vi "Koinzidenzschaltung.vi"() -> ()   [LabVIEW 2024]
panel:
  in  "Abbrechen":bool
  in  "Measunring Time (ms)":dbl max=0.0 step=10.0
  in  "StepSize (mV)":dbl max=0.0 step=10.0
  in  "Stop Value (mV)":dbl max=0.0 step=10.0
  out "Current Value":dbl
  in  "Start Value (mV)":dbl max=0.0 step=10.0
  out "Versoion":string
  out "NemBox ID":string
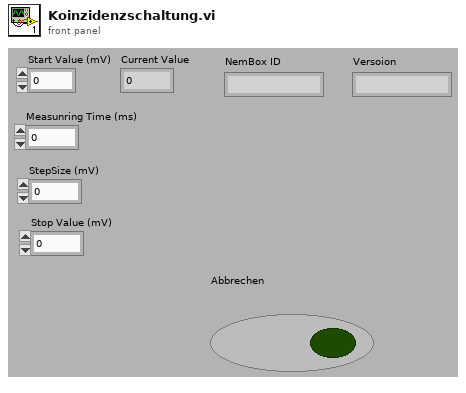
[diagram p1: front panel]
types:
  T1 = enum16{"Connect", "Get IN", "Write Threshold", "Write Hysteresis", "Write Stretch"}
  T2 = enum16{"Connect", "Set A", "Set B", "Set C", "Set D", "Set E", "Set F", "Set G", "Set H", "Get AND", "Read Counter", "Clear Counter"}
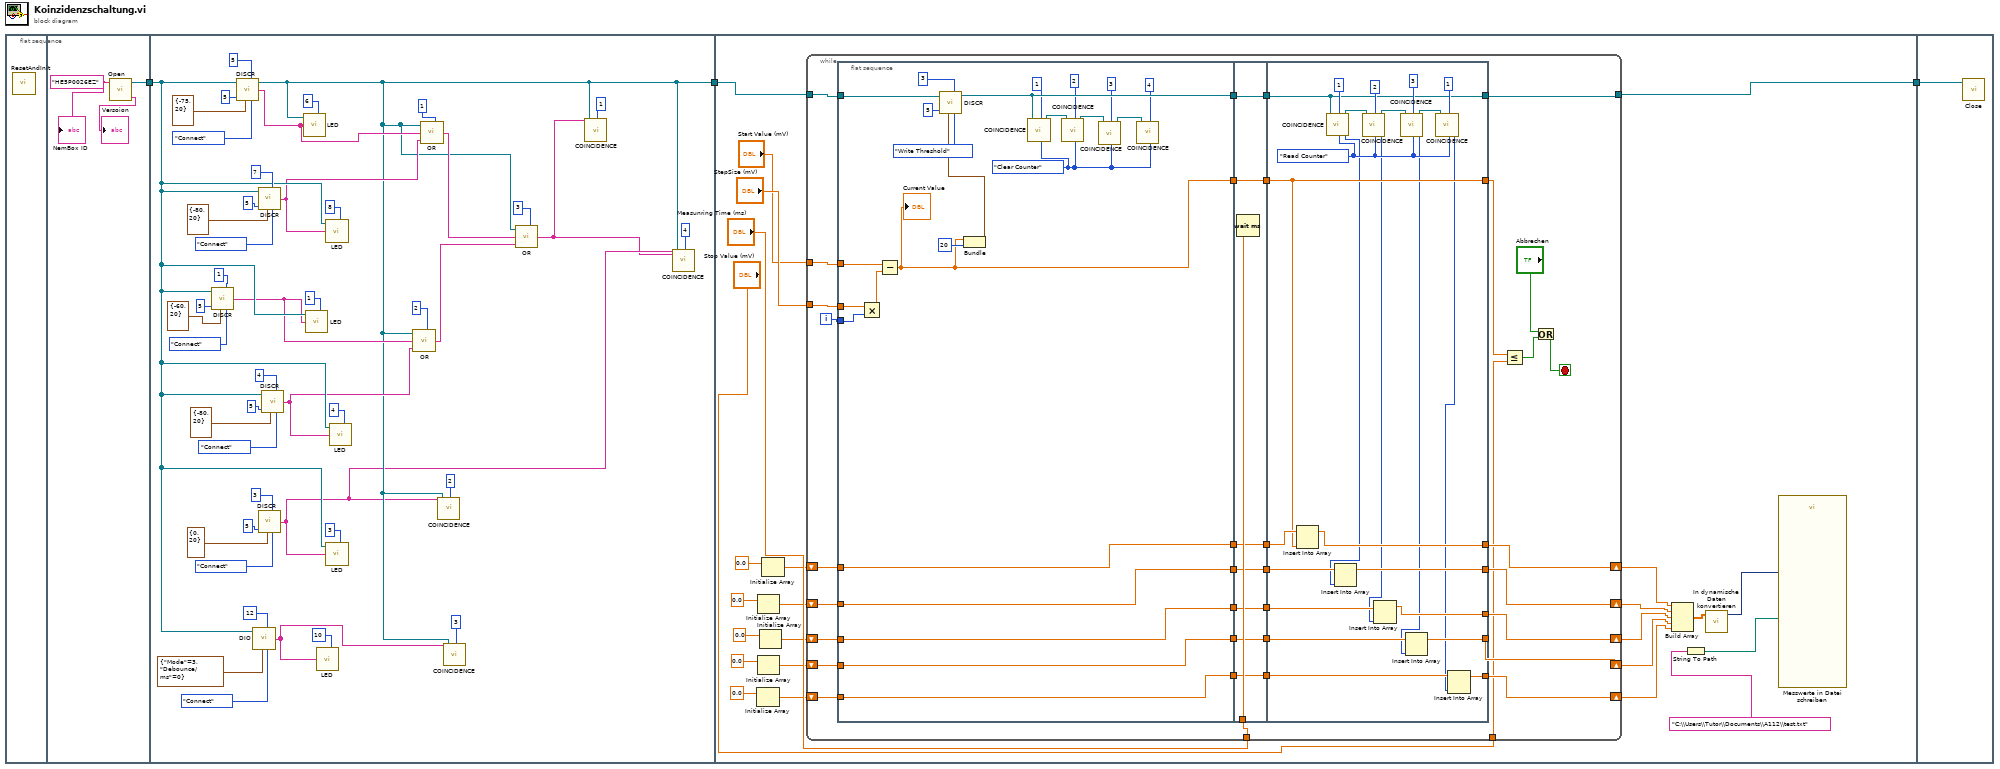
[diagram p0: block diagram]
diagram:
  n1 = flat-sequence {
    tunnel: [w6] -> w3
    tunnel: w3 -> [w25]
    tunnel: [w14] -> w2
    tunnel: w2 -> [w78]
    tunnel: [w63] -> w1
    tunnel: w1 -> [w171]
    frame #0 {
      n2 = call <userlib>:"ResetAndInit.vi"() -> ()  [unwired: 1 out]
    }
    frame #1 {
      w5 = "HE5P0026EZ"
      n3 = call <userlib>:"Open.vi"("USB_LogicBox"=w5) -> ("USB Out"=w6:refnum<visa-resource-name>, "Version"=→"Versoion":string)  [unwired: 1 in, 6 out]
      "NemBox ID" <- w5
    }
    frame #2 {
      n4 = call <userlib>:"DISCR.vi"("USB In"=w25, "Stretch/10ns"=u8 5, "Params"=cluster{i32, i32} {-60, 20} ("Schwelle"), "DISCR#"=1, "Function"=T1."Connect") -> ("DISCR"=w20:string)  [unwired: 4 out]
      n5 = call <userlib>:"DISCR.vi"("USB In"=w25, "Stretch/10ns"=u8 5, "Params"=cluster{i32, i32} {-75, 20} ("Schwelle"), "DISCR#"=u8 5, "Function"=T1."Connect") -> ("USB Out"=w14:refnum<visa-resource-name>, "DISCR"=w24:string)  [unwired: 3 out]
      n6 = call <userlib>:"DIO.vi"("USB In"=w25, "Params"=cluster{"Mode":u8, "Debounce/ms":u8} {"Mode"=3, "Debounce/ms"=0}, "DIO#"=12, "Function"=enum16{"Connect", "Set DO", "Get DI"}."Connect") -> ("DI"=w12:string)  [unwired: 1 in, 4 out]
      n7 = call <userlib>:"DISCR.vi"("USB In"=w25, "Stretch/10ns"=u8 5, "Params"=cluster{i32, i32} {-80, 20} ("Schwelle"), "DISCR#"=u8 7, "Function"=T1."Connect") -> ("DISCR"=w23:string)  [unwired: 4 out]
      n8 = call <userlib>:"DISCR.vi"("Stretch/10ns"=u8 5, "Params"=cluster{i32, i32} {0, 20} ("Schwelle"), "DISCR#"=u8 3, "Function"=T1."Connect") -> ("DISCR"=w11:string)  [unwired: 1 in, 4 out]
      n9 = call <userlib>:"DISCR.vi"("USB In"=w25, "Stretch/10ns"=u8 5, "Params"=cluster{i32, i32} {-80, 20} ("Schwelle"), "DISCR#"=u8 4, "Function"=T1."Connect") -> ("DISCR"=w19:string)  [unwired: 4 out]
      n10 = call <userlib>:"LED.vi"("USB In"=w14, "STATE"=w24, "LED#"=u8 6) -> ()  [unwired: 6 in, 1 out]
      n11 = call <userlib>:"LED.vi"("USB In"=w25, "STATE"=w20, "LED#"=u8 1) -> ()  [unwired: 6 in, 1 out]
      n12 = call <userlib>:"LED.vi"("STATE"=w12, "LED#"=u8 10) -> ()  [unwired: 7 in, 1 out]
      n13 = call <userlib>:"LED.vi"("USB In"=w25, "STATE"=w23, "LED#"=u8 8) -> ()  [unwired: 6 in, 1 out]
      n14 = call <userlib>:"LED.vi"("USB In"=w25, "STATE"=w11, "LED#"=u8 3) -> ()  [unwired: 6 in, 1 out]
      n15 = call <userlib>:"LED.vi"("USB In"=w25, "STATE"=w19, "LED#"=u8 4) -> ()  [unwired: 6 in, 1 out]
      n16 = call <userlib>:"OR.vi"("USB In"=w14, "A"=w20, "B"=w19, "LOGIC#"=u8 2) -> ("OR"=w17:string)  [unwired: 4 in, 1 out]
      n17 = call <userlib>:"OR.vi"("USB In"=w14, "A"=w24, "B"=w23, "LOGIC#"=u8 1) -> ("OR"=w18:string)  [unwired: 4 in, 1 out]
      n18 = call <userlib>:"COINCIDENCE.vi"("A"=w11, "USB In"=w14, "CC#"=u8 2) -> ()  [unwired: 8 in, 17 out]
      n19 = call <userlib>:"COINCIDENCE.vi"("A"=w12, "USB In"=w14, "CC#"=u8 3) -> ()  [unwired: 8 in, 17 out]
      n20 = call <userlib>:"OR.vi"("USB In"=w14, "A"=w18, "B"=w17, "LOGIC#"=u8 3) -> ("OR"=w7:string)  [unwired: 4 in, 1 out]
      n21 = call <userlib>:"COINCIDENCE.vi"("A"=w7, "USB In"=w14, "CC#"=u8 1) -> ()  [unwired: 8 in, 17 out]
      n22 = call <userlib>:"COINCIDENCE.vi"("A"=w11, "B"=w7, "USB In"=w14, "CC#"=u8 4) -> ()  [unwired: 7 in, 17 out]
    }
    frame #3 {
      n23 = Initialize Array(0.0 ("Start Value 2")) -> (w65:dbl[])  [unwired: 1 out]
      n24 = Initialize Array(0.0 ("Start Value 2")) -> (w68:dbl[])  [unwired: 1 out]
      n25 = Initialize Array(0.0 ("Start Value 2")) -> (w66:dbl[])  [unwired: 1 out]
      n26 = Initialize Array(0.0 ("Start Value 2")) -> (w67:dbl[])  [unwired: 1 out]
      n27 = Initialize Array(0.0 ("Start Value 2")) -> (w69:dbl[])  [unwired: 1 out]
      n28 = while {
        tunnel: w78 -> [w112]
        tunnel: [w111] -> w63
        tunnel: "StepSize (mV)" -> [w110]
        tunnel: "Start Value (mV)" -> [w109]
        tunnel: "Measunring Time (ms)" -> [w106]
        shift-right: [w99] -> w57
        shift-left: w68 -> [w98]
        shift-right: [w100] -> w58
        shift-left: w69 -> [w103]
        shift-right: [w94] -> w56
        shift-left: w67 -> [w95]
        shift-right: [w90] -> w55
        shift-left: w66 -> [w91]
        shift-right: [w86] -> w54
        shift-left: w65 -> [w87]
        tunnel: "Stop Value (mV)" -> [w82]
        i -> [w113]
        stop <- w80 stop-if-true
        n29 = flat-sequence {
          tunnel: w113 -> [w131]
          tunnel: w112 -> [w133]
          tunnel: w110 -> [w132]
          tunnel: w109 -> [w130]
          tunnel: [w128] -> w108
          tunnel: [w120] -> w104
          tunnel: w103 -> [w120]
          tunnel: [w119] -> w101
          tunnel: w98 -> [w119]
          tunnel: [w118] -> w96
          tunnel: w95 -> [w118]
          tunnel: [w117] -> w92
          tunnel: w91 -> [w117]
          tunnel: [w116] -> w88
          tunnel: w87 -> [w116]
          tunnel: [w115] -> w84
          tunnel: w108 -> [w146]
          tunnel: [w146] -> w107
          tunnel: w106 -> [w145]
          tunnel: [w144] -> w105
          tunnel: w104 -> [w144]
          tunnel: [w143] -> w102
          tunnel: w101 -> [w143]
          tunnel: [w142] -> w97
          tunnel: w96 -> [w142]
          tunnel: [w141] -> w93
          tunnel: w92 -> [w141]
          tunnel: [w140] -> w89
          tunnel: w88 -> [w140]
          tunnel: [w139] -> w85
          tunnel: w84 -> [w139]
          tunnel: [w166] -> w111
          tunnel: w107 -> [w166]
          tunnel: w105 -> [w162]
          tunnel: w102 -> [w161]
          tunnel: [w160] -> w100
          tunnel: [w159] -> w99
          tunnel: w97 -> [w158]
          tunnel: [w157] -> w94
          tunnel: w93 -> [w156]
          tunnel: [w155] -> w90
          tunnel: w89 -> [w154]
          tunnel: [w153] -> w86
          tunnel: [w151] -> w83
          tunnel: w85 -> [w151]
          frame #0 {
            w114 = T2."Clear Counter"
            n30 = Multiply(x=w132, y=w131) -> (x*y=w129:dbl)
            n31 = Subtract(x=w130, y=w129) -> (x-y=w115:dbl)
            "Current Value" <- w115
            n32 = Bundle(w115, 20) -> (w135:cluster{dbl, i32})  [unwired: 1 out]
            n33 = call <userlib>:"DISCR.vi"("USB In"=w133, "Stretch/10ns"=u8 5, "Params"=w135, "DISCR#"=3, "Function"=T1."Write Threshold") -> ("USB Out"=w128:refnum<visa-resource-name>)  [unwired: 4 out]
            n34 = call <userlib>:"COINCIDENCE.vi"("USB In"=w128, "CC#"=u8 1, "Function"=w114) -> ("USB Out"=w123:refnum<visa-resource-name>)  [unwired: 8 in, 16 out]
            n35 = call <userlib>:"COINCIDENCE.vi"("USB In"=w123, "CC#"=u8 2, "Function"=w114) -> ("USB Out"=w122:refnum<visa-resource-name>)  [unwired: 8 in, 16 out]
            n36 = call <userlib>:"COINCIDENCE.vi"("USB In"=w122, "CC#"=u8 3, "Function"=w114) -> ("USB Out"=w121:refnum<visa-resource-name>)  [unwired: 8 in, 16 out]
            n37 = call <userlib>:"COINCIDENCE.vi"("USB In"=w121, "CC#"=u8 4, "Function"=w114) -> ()  [unwired: 8 in, 17 out]
          }
          frame #1 {
            n38 = Wait (ms)(milliseconds to wait=w145) -> ()  [unwired: 1 out]
          }
          frame #2 {
            w152 = T2."Read Counter"
            n39 = Insert Into Array(array=w162, new element=w151) -> (w160:dbl[])  [unwired: 1 in]
            n40 = call <userlib>:"COINCIDENCE.vi"("USB In"=w166, "CC#"=u8 1, "Function"=w152) -> ("USB Out"=w163:refnum<visa-resource-name>, "Counter"=w150:u32)  [unwired: 8 in, 15 out]
            n41 = Insert Into Array(array=w161, new element=w150) -> (w159:dbl[])  [unwired: 1 in]
            n42 = call <userlib>:"COINCIDENCE.vi"("USB In"=w163, "CC#"=u8 2, "Function"=w152) -> ("USB Out"=w164:refnum<visa-resource-name>, "Counter"=w149:u32)  [unwired: 8 in, 15 out]
            n43 = Insert Into Array(array=w158, new element=w149) -> (w157:dbl[])  [unwired: 1 in]
            n44 = call <userlib>:"COINCIDENCE.vi"("USB In"=w164, "CC#"=u8 3, "Function"=w152) -> ("USB Out"=w165:refnum<visa-resource-name>, "Counter"=w148:u32)  [unwired: 8 in, 15 out]
            n45 = Insert Into Array(array=w156, new element=w148) -> (w155:dbl[])  [unwired: 1 in]
            n46 = call <userlib>:"COINCIDENCE.vi"("USB In"=w165, "CC#"=u8 1, "Function"=w152) -> ("Counter"=w147:u32)  [unwired: 8 in, 16 out]
            n47 = Insert Into Array(array=w154, new element=w147) -> (w153:dbl[])  [unwired: 1 in]
          }
        }
        n48 = Less Or Equal?(x=w83, y=w82) -> (x <= y?=w81:bool)
        n49 = Or(x="Abbrechen", y=w81) -> (x .or. y?=w80:bool)
      }
      n50 = Build Array(w58, w57, w56, w55, w54) -> (w59:dbl[][])
      n51 = String To Path(string="C:\\Users\\Tutor\\Documents\\A112\\test.txt") -> (path=w61:path)
      n52 = call "In dynamische Daten konvertieren"("2D Array"=w59) -> ("Dynamic Data Type"=w60:dynamicdata)  [unwired: 3 out]
      n53 = call "Messwerte in Datei schreiben"("Signals"=w60, "Filename"=w61) -> ()  [unwired: 15 in, 3 out]
    }
    frame #4 {
      n54 = call <userlib>:"Close.vi"("USB In"=w171) -> ()  [unwired: 1 in, 8 out]
    }
  }
